vi "SetDataFlowMap.vi"(8 "error in (no error)":errorcluster, 10 "type":T1, 11 "Dataflow script":string[](array[string])) -> (0 "error out":errorcluster)   [LabVIEW 2017, in "DataFlow.lvlib"]
uses:
  <vilib>/addons/InsightCM/Devices/Shared/Common/DataFlow/DataFlow.lvlib
  <vilib>/addons/InsightCM/Devices/Shared/Common/DataFlow/controls/Type.ctl
  <vilib>/addons/PointValueMap/subVIs/Point_Write_variant.vi
  <vilib>/addons/InsightCM/Utilities/GlobalConfiguration/GlobalConfiguration.lvlib
  <vilib>/addons/PointValueMap/PointValueMap.lvlib
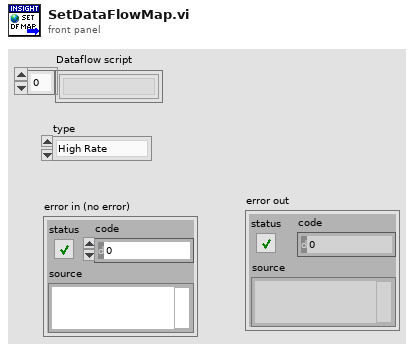
[diagram p1: front panel]
types:
  T1 = typedef "DataFlow.lvlib/Type.ctl" = enum16{"High Rate", "Low Rate", "Burst Mode"}
  T2 = typedef "PointValueMap.lvlib/PointMap.ctl" = refnum<data-value>
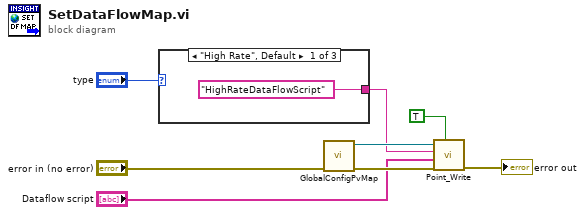
[diagram p0: block diagram]
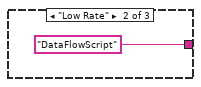
[diagram p2: hidden frame]
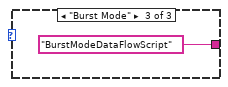
[diagram p3: hidden frame]
diagram:
  n1 = case shown="\"High Rate\", Default" "type" {
    tunnel: ["HighRateDataFlowScript" ("Name") "DataFlowScript" ("Name") "BurstModeDataFlowScript" ("Name")] -> w1
    frame "High Rate", Default {
    }
    frame "Low Rate" {
    }
    frame "Burst Mode" {
    }
  }
  n2 = call <vilib>:"GlobalConfigPvMap.vi"("error in (no error)"="error in (no error)") -> ("error out"=w7:errorcluster, "global configuration map"=w6:T2)  [unwired: 9 in]
  n3 = call-poly <vilib>:"Point_Write.vi"("Auto Create?"=TRUE, "Error In"=w7, "Value"="Dataflow script", "Tag"=w1, "Map"=w6) -> ("Error Out"=→"error out":errorcluster)  [unwired: 5 in, 1 out]
